vi "replace dot with coma if loc dez poin used.vi"(8 "error in (no error)":errorcluster, 11 "String in":string) -> (0 "error out":errorcluster, 3 "String out":string)   [LabVIEW 2009, in "POLARIS BME DG.lvlib"]
uses:
  POLARIS BME DG.lvlib
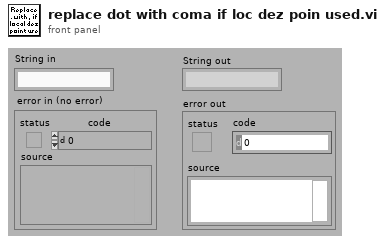
[diagram p1: front panel]
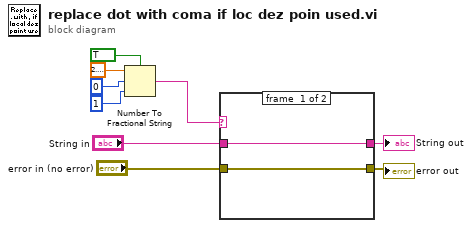
[diagram p0: block diagram]
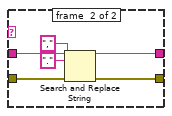
[diagram p2: hidden frame]
diagram:
  n1 = Number To Fractional String(use system decimal point (T)=TRUE, number=2.718281828459045, width (-)=i16 0, precision (6)=i16 1) -> (F-format string=w1:string)
  n2 = case shown="\"2,7\"" w1 {
    tunnel: "error in (no error)" -> [w10 w17]
    tunnel: [w10 w16] -> w2
    tunnel: "String in" -> [w11 w15]
    tunnel: [w11 w12] -> w3
    frame #0 {
    }
    frame #1 {
      n3 = Search and Replace String(input string=w15, search string=".", replace string="," ("replace string (\"\")"), error in=w17) -> (result string=w12:string, error out=w16:errorcluster)  [unwired: 4 in, 2 out]
    }
  }
  "String out" <- w3
  "error out" <- w2
